vi "set_pixel_frequency.vi"(8 "error in (no error)":errorcluster, 10 "pixel frequency":dbl[unit], 11 "FPGAWrapperDL090211Galvo_grabber in":refnum<class "FPGAWrapperDL090211Galvo.lvclass">) -> (0 "error out":errorcluster, 3 "FPGAWrapperDL090211Galvo_grabber out":refnum<class "FPGAWrapperDL090211Galvo.lvclass">)   [LabVIEW 2010, in "FPGAWrapperDL090211Galvo.lvclass"]
uses:
  FPGAWrapperDL090211Galvo.lvclass
  GenericFPGAWrapper/GenericFPGAWrapper/GenericFPGAWrapper.lvclass
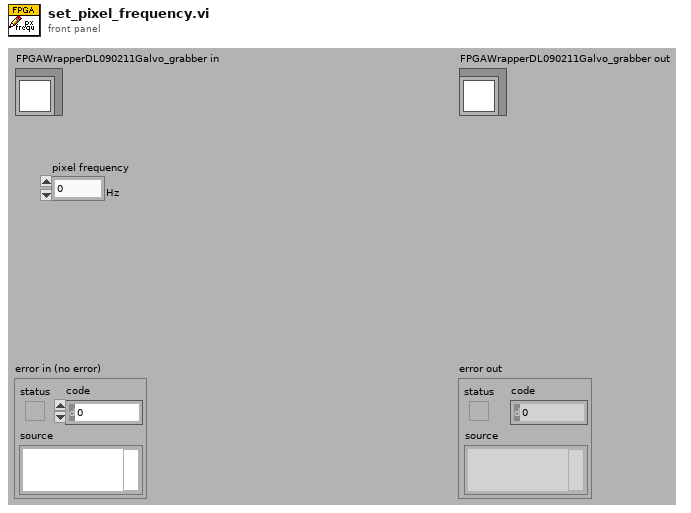
[diagram p1: front panel]
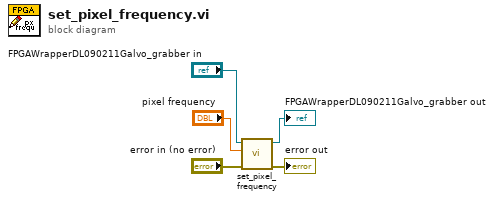
[diagram p0: block diagram]
diagram:
  n1 = call-parent "set_pixel_frequency.vi"("error in (no error)"="error in (no error)", "pixel frequency"="pixel frequency", "GenericFPGAWrapper in"="FPGAWrapperDL090211Galvo_grabber in") -> ("error out"=→"error out":errorcluster, "GenericFPGAWrapper out"=→"FPGAWrapperDL090211Galvo_grabber out":refnum<class "FPGAWrapperDL090211Galvo.lvclass">)  [unwired: 7 in]
